vi "_Add Sheet.vi"(8 "error in":errorcluster, 10 "SheetName":string, 11 "SpreadsheetDoc in":refnum<k24>) -> (0 "error out":errorcluster, 1 "Sheet Index":i32, 2 "Sheet":refnum<k24>, 3 "SpreadsheetDoc out":refnum<k24>)   [LabVIEW 2019, in "Open Xml.lvlib"]
uses:
  Open Xml.lvlib
  D:/git/Open-Xml-LabVIEW/Source/DocumentFormat.OpenXml.dll
  DocumentFormat.OpenXml.dll
  D:/git/Open-Xml-LabVIEW/Source/DocumentFormat.OpenXml.Framework.dll
  DocumentFormat.OpenXml.Framework.dll
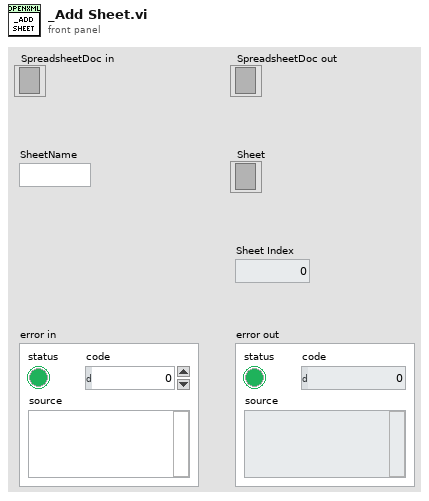
[diagram p1: front panel]
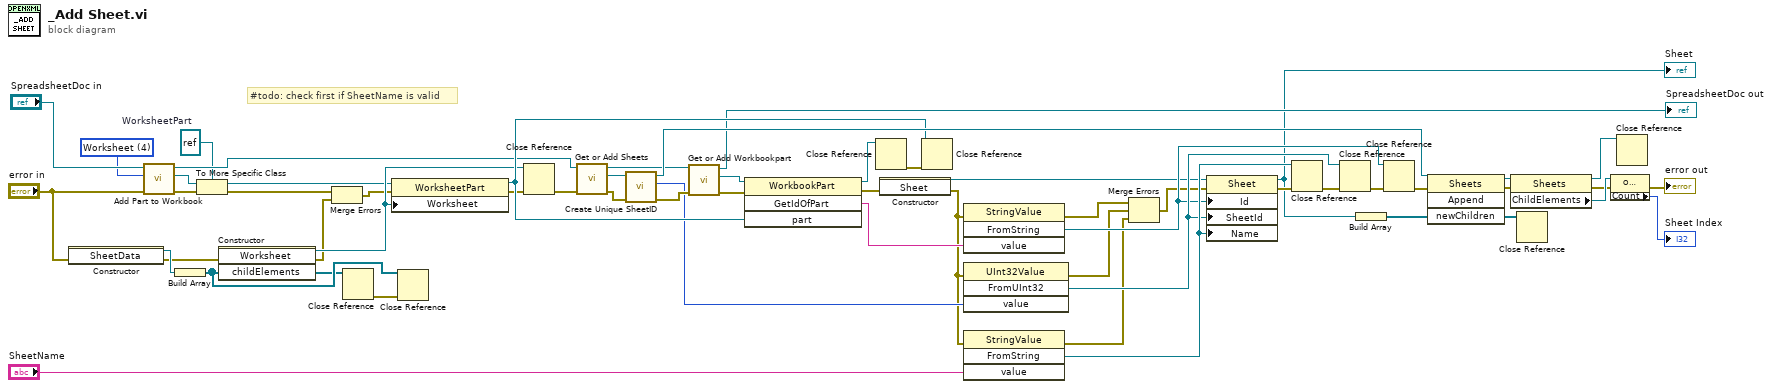
[diagram p0: block diagram]
diagram:
  w6 = 4 items=["Connections", "PivotTableCacheDefinition", "PivotTableCacheRecords", "SharedStringTable", "Worksheet", "WorkbookStyles"] ("PartType")
  w22 = refnum<k24> refnum  # WorksheetPart
  # "#todo: check first if SheetName is valid"
  n1 = constructor class="SheetData"(error in="error in") -> (reference out=w21:refnum<k24>, error out=w20:errorcluster)  [unwired: 2 in, 1 out]
  n2 = call "Add Part to Workbook.vi"("error in"="error in", "PartType"=w6, "SpreadsheetDoc in"="SpreadsheetDoc in") -> ("error out"=w27:errorcluster, "OpenXmlPart"=w19:refnum<k24>, "SpreadsheetDoc out"=w35:refnum<k24>)  [unwired: 6 in]
  n3 = Build Array(w21) -> (w26:refnum<k24>[])
  n4 = To More Specific Class(target class=w22, reference=w19, error in=w27) -> (specific class reference=w23:refnum<k24>, error out=w28:errorcluster)
  n5 = constructor class="Worksheet"(error in=w20, "childElements"=w26) -> (reference out=w33:refnum<k24>, error out=w31:errorcluster, "childElements"=w25:refnum<k24>[])  [unwired: 2 in, 1 out]
  n6 = Merge Errors(w28, w31) -> (w30:errorcluster)
  n7 = Close Reference(reference=w25) -> (error out=w24:errorcluster)  [unwired: 1 in]
  n8 = property on="New WorksheetPart" class="WorksheetPart"(reference=w23, error in=w30, "Worksheet"=w33) -> (reference out=w52:refnum<k24>, error out=w32:errorcluster)
  n9 = Close Reference(reference=w26, error in (no error)=w24) -> ()  [unwired: 1 out]
  n10 = Close Reference(reference=w33, error in (no error)=w32) -> (error out=w34:errorcluster)
  n11 = call "Get or Add Sheets.vi"("error in"=w34, "SpreadsheetDoc in"=w35) -> ("error out"=w55:errorcluster, "Sheets"=w53:refnum<k24>, "SpreadsheetDoc out"=w38:refnum<k24>)  [unwired: 7 in]
  n12 = call "Create Unique SheetID.vi"("error in"=w55, "Sheets in"=w53) -> ("error out"=w56:errorcluster, "Unique SheetID"=w41:u32, "Sheets out"=w54:refnum<k24>)  [unwired: 7 in]
  n13 = call "Get or Add Workbookpart.vi"("error in"=w56, "SpreadsheetDoc in"=w38) -> ("error out"=w37:errorcluster, "WorkbookPart"=w36:refnum<k24>, "SpreadsheetDoc out"=→"SpreadsheetDoc out":refnum<k24>)  [unwired: 7 in]
  n14 = invoke class="WorkbookPart" method="GetIdOfPart"(reference=w36, error in=w37, "part"=w52) -> (reference out=w57:refnum<k24>, error out=w14:errorcluster, "GetIdOfPart"=w40:string)  [unwired: 1 in, 1 out]
  n15 = Close Reference(reference=w57) -> (error out=w13:errorcluster)  [unwired: 1 in]
  n16 = constructor class="Sheet"(error in=w14) -> (reference out=w39:refnum<k24>, error out=w5:errorcluster)  [unwired: 2 in, 1 out]
  n17 = Close Reference(reference=w52, error in (no error)=w13) -> ()  [unwired: 1 out]
  n18 = invoke class="StringValue" method="FromString"(error in=w5, "value"=w40) -> (error out=w2:errorcluster, "FromString"=w43:refnum<k24>)  [unwired: 2 in, 2 out]
  n19 = invoke class="UInt32Value" method="FromUInt32"(error in=w5, "value"=w41) -> (error out=w3:errorcluster, "FromUInt32"=w45:refnum<k24>)  [unwired: 2 in, 2 out]
  n20 = invoke class="StringValue" method="FromString"(error in=w5, "value"="SheetName") -> (error out=w4:errorcluster, "FromString"=w48:refnum<k24>)  [unwired: 2 in, 2 out]
  n21 = Merge Errors(w2, w3, w4) -> (w1:errorcluster)
  n22 = property class="Sheet"(reference=w39, error in=w1, "Id"=w43, "SheetId"=w45, "Name"=w48) -> (reference out=w15:refnum<k24>, error out=w42:errorcluster)
  "Sheet" <- w15
  n23 = Close Reference(reference=w48, error in (no error)=w42) -> (error out=w47:errorcluster)
  n24 = Close Reference(reference=w45, error in (no error)=w47) -> (error out=w44:errorcluster)
  n25 = Build Array(w15) -> (w17:refnum<k24>[])
  n26 = Close Reference(reference=w43, error in (no error)=w44) -> (error out=w49:errorcluster)
  n27 = invoke class="Sheets" method="Append"(reference=w54, error in=w49, "newChildren"=w17) -> (reference out=w12:refnum<k24>, error out=w50:errorcluster, "newChildren"=w18:refnum<k24>[])  [unwired: 1 in, 1 out]
  n28 = property class="Sheets"(reference=w12, error in=w50) -> (reference out=w11:refnum<k24>, error out=w8:errorcluster, "ChildElements"=w10:refnum<k24>)
  n29 = Close Reference(reference=w18) -> ()  [unwired: 1 in, 1 out]
  n30 = property class="OpenXmlElementList"(reference=w10, error in=w8) -> (error out=→"error out":errorcluster, "Count"=→"Sheet Index":i32)  [unwired: 1 out]
  n31 = Close Reference(reference=w11) -> ()  [unwired: 1 in, 1 out]
